vi "Get Section Names.vi"(8 "error in (no error)":errorcluster, 11 "refnum":T1) -> (0 "error out":errorcluster, 1 "plugin names":string[](array[string]), 3 "refnum out":T1)   [LabVIEW 2017]
doc: "Gets the names of all sections from the configuration data identified by <B>refnum</B>."
uses:
  DSFConfig.lvlib
  DSF Config Data RefNum.ctl
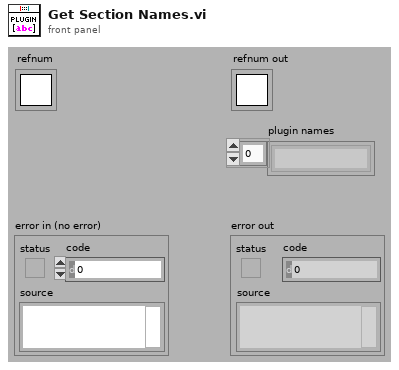
[diagram p1: front panel]
types:
  T1 = typedef "DSFConfig.lvlib/DSF Config Data RefNum.ctl" = refnum<k1>
  T2 = typedef "DSFConfig.lvlib/Config Queue.ctl" = refnum<queue>
  T3 = typedef "DSFConfig.lvlib/Config Data.ctl" = cluster{"dsf configuration":T4, "path":path, "dirty":bool}
  T4 = typedef "DSFConfig.lvlib/DSF Config.ctl" = cluster{"dsf":T5, "configuration":T5, "plugins":T6[], "groups":T9[], "transfers":T11[], "channels":T13[], "settings":T15[]}
  T5 = typedef "DSFConfig.lvlib/Version Info.ctl" = cluster{"major":u32, "minor":u32, "fix":u32, "build":string}
  T6 = typedef "DSFConfig.lvlib/DSF Plugin.ctl" = cluster{"id":string, "values":T7}
  T7 = typedef "DSFConfig.lvlib/DSF Plugin Info.ctl" = cluster{"type":string, "timing":T8, "group ids":string[], "settings id":string}
  T8 = typedef "DSFConfig.lvlib/DSF Timing Info.ctl" = cluster{"decimation":i32, "offset":i32}
  T9 = typedef "DSFConfig.lvlib/DSF Group.ctl" = cluster{"id":string, "values":T10}
  T10 = typedef "DSFConfig.lvlib/DSF Group Info.ctl" = cluster{"direction":i32, "timing":T8, "transfer ids":string[], "settings id":string}
  T11 = typedef "DSFConfig.lvlib/DSF Transfer.ctl" = cluster{"id":string, "values":T12}
  T12 = typedef "DSFConfig.lvlib/DSF Transfer Info.ctl" = cluster{"byte order":i32, "channel ids":string[], "settings id":string}
  T13 = typedef "DSFConfig.lvlib/DSF Channel.ctl" = cluster{"id":string, "values":T14}
  T14 = typedef "DSFConfig.lvlib/DSF Channel Info.ctl" = cluster{"count":i32, "offset":i32, "data type":i32, "resource path":string, "settings id":string}
  T15 = typedef "DSFConfig.lvlib/DSF Settings.ctl" = cluster{"id":string, "values":T16}
  T16 = typedef "DSFConfig.lvlib/DSF Settings Info.ctl" = cluster{"key":string, "value":string}[]
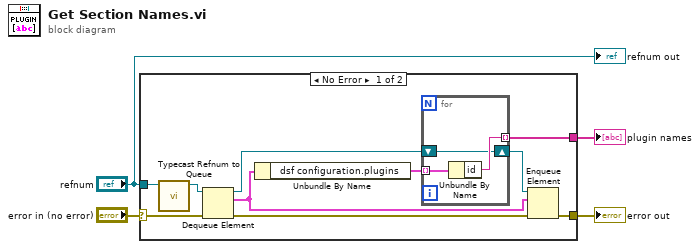
[diagram p0: block diagram]
diagram:
  n1 = case shown="No Error" "error in (no error)" {
    selector: "error in (no error)" -> [w10 w18]
    tunnel: [w13 _] -> w2
    tunnel: [w8 w18] -> w3
    tunnel: "refnum" -> [w12 _]
    frame No Error {
      n2 = call "Typecast Refnum to Queue.vi"("refnum in"=w12) -> ("queue out"=w14:T2)  [unwired: 10 in]
      n3 = Dequeue Element(queue=w14, error in (no error)=w10) -> (queue out=w7:T2, element=w5:T3, error out=w9:errorcluster)  [unwired: 1 in, 1 out]
      n4 = Unbundle By Name(w5) -> ("dsf configuration.plugins"=w11:T6[])
      n5 = for {
        tunnel: w11 -> [w16] mode=indexing
        tunnel: [w17] -> w13 mode=indexing
        shift-right: [w15] -> w6
        shift-left: w7 -> [w15]
        n6 = Unbundle By Name(w16) -> ("id"=w17:string)
      }
      n7 = Enqueue Element(queue=w6, element=w5, error in (no error)=w9) -> (error out=w8:errorcluster)  [unwired: 1 in, 2 out]
    }
    frame Error {
    }
  }
  "error out" <- w3
  "plugin names" <- w2
  "refnum out" <- "refnum"
